vi "Add Date Scrubber.vi"() -> ()   [LabVIEW 2020, in "Approval Tests.lvlib"]
doc: "Drops everything needed to filter out dates."
uses:
  Approval Tests.lvlib
  Options/Options.lvclass
  Date Scrubber/Date Scrubber.lvclass
  C:/Users/SAS/Desktop/ApprovalTests.LabVIEW/Source/Approval Tests/Scrubber/Scrubber.lvclass
  Options/Write Add Scrubber.vi
panel:
  out "Found?":bool
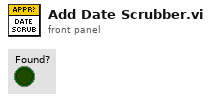
[diagram p1: front panel]
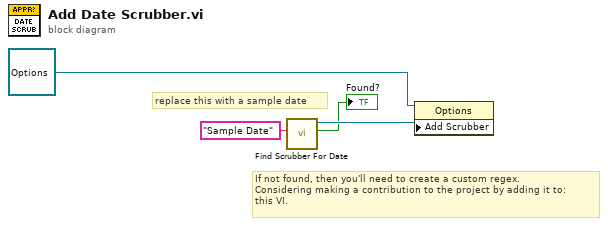
[diagram p0: block diagram]
diagram:
  # "If not found, then you'll need to create a custom regex.\nConsidering making a contribution to the project by adding it to:\nthis VI."
  # "replace this with a sample date"
  n1 = call "Find Scrubber For Date.vi"("Sample Date"="Sample Date") -> ("Found?"=→"Found?":bool, "Date Scrubber out"=w3:refnum<class "Date Scrubber.lvclass">)  [unwired: 8 in, 1 out]
  n2 = property class="Options"(reference=refnum<class "Options.lvclass"> refnum ("Approval Tests.lvlib:Options"), "Add Scrubber"=w3) -> ()  [unwired: 1 in, 2 out]
